vi "SetRemote.vi"(4 "error in":errorcluster, 5 "connection ID":refnum<k5>) -> (1 "error out":errorcluster, 2 "connection ID out":refnum<k5>, 3 "Answer":bool)   [LabVIEW 2015]
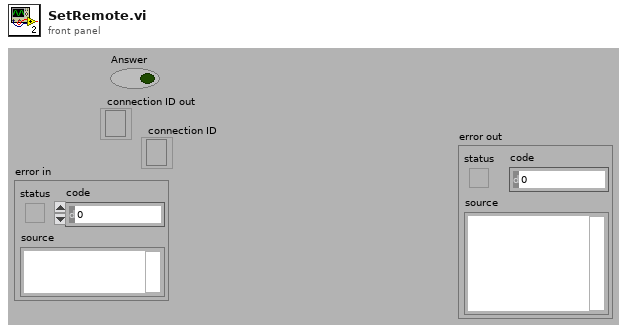
[diagram p1: front panel]
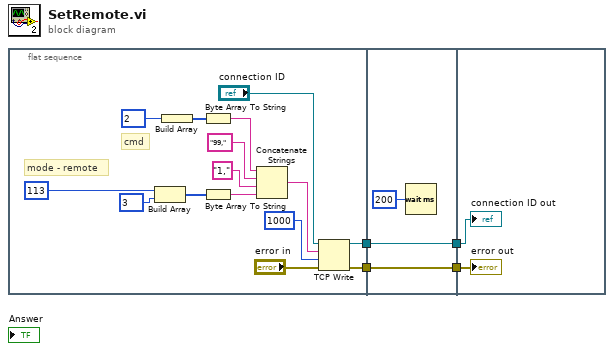
[diagram p0: block diagram]
diagram:
  n1 = flat-sequence {
    tunnel: [w16] -> w3
    tunnel: [w15] -> w1
    tunnel: [w22] -> w4
    tunnel: w3 -> [w22]
    tunnel: [w21] -> w2
    tunnel: w1 -> [w21]
    tunnel: w4 -> [w23]
    tunnel: w2 -> [w24]
    frame #0 {
      # "cmd"
      # "mode - remote"
      n2 = Build Array(u8 113 ("y"), u8 3 ("y")) -> (w8:u8[])
      n3 = Build Array(u8 2 ("y")) -> (w12:u8[])
      n4 = Byte Array To String(unsigned byte array=w12) -> (string=w11:string)
      n5 = Byte Array To String(unsigned byte array=w8) -> (string=w5:string)
      n6 = Concatenate Strings(w11, "99," ("string"), "1," ("string"), w5) -> (w7:string)
      n7 = TCP Write(connection ID="connection ID", data in=w7, error in (no error)="error in", 9:1000 ("timeout ms (25000)")) -> (connection ID out=w16:refnum<k5>, error out=w15:errorcluster)  [unwired: 1 out]
    }
    frame #1 {
      n8 = Wait (ms)(milliseconds to wait=u32 200) -> ()  [unwired: 1 out]
    }
    frame #2 {
      "connection ID out" <- w23
      "error out" <- w24
    }
  }
